vi "Timestamp to Value.vi"(10 "name":string, 11 "timestamp":dbl) -> (2 "value":dbl, 3 "timestamp (dup)":dbl)   [LabVIEW 2021, in "RocketPlotDemo.lvlib"]
uses:
  RocketPlotDemo.lvlib
  Demo Names.ctl
  <vilib>/ptbypt/NI_PtbyPt.lvlib
  <userlib>/_OpenG.lib/lvdata/lvdata.llb/openg_variant.lvlib
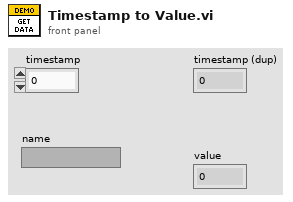
[diagram p1: front panel]
types:
  T1 = typedef "RocketPlotDemo.lvlib/Demo Names.ctl" = enum16{"Sine Wave", "Triangle Wave", "Sawtooth Wave", "Square Wave", "Uniform Noise", "Periodic Noise", "White Noise"}
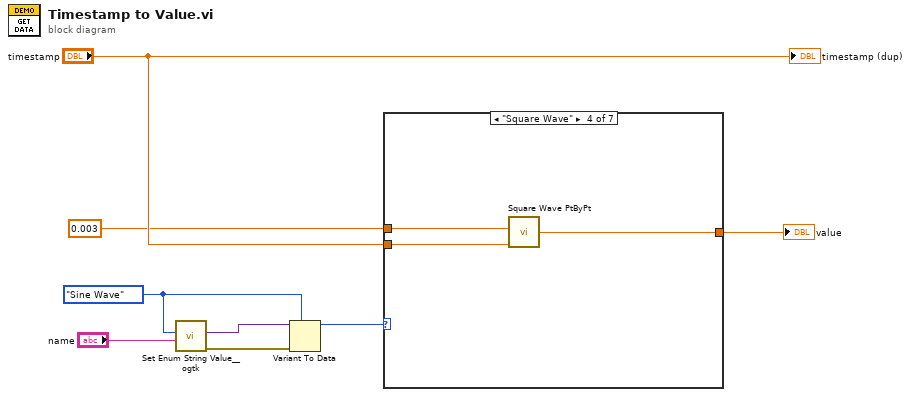
[diagram p0: block diagram]
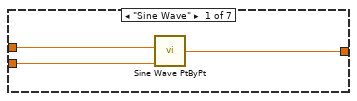
[diagram p2: hidden frame]
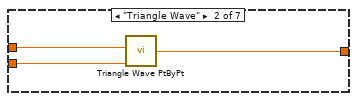
[diagram p3: hidden frame]
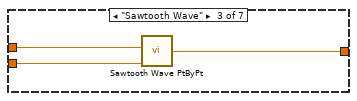
[diagram p4: hidden frame]
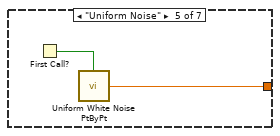
[diagram p5: hidden frame]
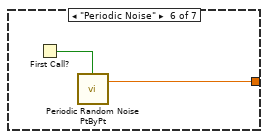
[diagram p6: hidden frame]
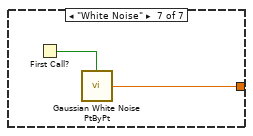
[diagram p7: hidden frame]
diagram:
  w3 = Demo_Names."Sine Wave" ("channel")
  n1 = call <userlib>:"Set Enum String Value__ogtk.vi"("String Value"="name", "Default Enum Value"=w3) -> ("error out"=w4:errorcluster, "Enum"=w5:variant)  [unwired: 8 in]
  n2 = Variant To Data(error in=w4, type=w3, Variant=w5) -> (data=w1:T1)  [unwired: 1 out]
  n3 = case shown="\"Square Wave\"" w1 {
    tunnel: [w11 w13 w16 w19 w22 w24 w26] -> w8
    tunnel: "timestamp" -> [w10 w14 w17 w20 _ _ _]
    tunnel: 0.003 ("frequency") -> [w9 w12 w15 w18 _ _ _]
    frame "Sine Wave" {
      n4 = call <vilib>:"Sine Wave PtByPt.vi"("time"=w10, "frequency"=w9) -> ("sine wave"=w11:dbl)  [unwired: 2 in]
    }
    frame "Triangle Wave" {
      n5 = call <vilib>:"Triangle Wave PtByPt.vi"("time"=w14, "frequency"=w12) -> ("triangle wave"=w13:dbl)  [unwired: 2 in]
    }
    frame "Sawtooth Wave" {
      n6 = call <vilib>:"Sawtooth Wave PtByPt.vi"("time"=w17, "frequency"=w15) -> ("sawtooth wave"=w16:dbl)  [unwired: 2 in]
    }
    frame "Square Wave" {
      n7 = call <vilib>:"Square Wave PtByPt.vi"("frequency"=w18, "time"=w20) -> ("square wave"=w19:dbl)  [unwired: 3 in]
    }
    frame "Uniform Noise" {
      n8 = First Call?() -> (First Call?: T/F=w21:bool)
      n9 = call <vilib>:"Uniform White Noise PtByPt.vi"("initialize"=w21) -> ("uniform white noise"=w22:dbl)  [unwired: 2 in]
    }
    frame "Periodic Noise" {
      n10 = First Call?() -> (First Call?: T/F=w23:bool)
      n11 = call <vilib>:"Periodic Random Noise PtByPt.vi"("initialize"=w23) -> ("periodic random noise"=w24:dbl)  [unwired: 3 in, 1 out]
    }
    frame "White Noise" {
      n12 = First Call?() -> (First Call?: T/F=w25:bool)
      n13 = call <vilib>:"Gaussian White Noise PtByPt.vi"("initialize"=w25) -> ("Gaussian white noise"=w26:dbl)  [unwired: 2 in]
    }
  }
  "value" <- w8
  "timestamp (dup)" <- "timestamp"
